vi "Power Supply Initialize Chain.vi"(0 "reference in":refnum<class "Power Supply.lvclass">, 5 "Power Supply Chain VISA Resource":refnum<visa-resource-name>="Serial-Hub-1", 7 "Baud Rate":u16(ring)=3 items=["1200", "2400", "4800", "9600", "19200"], 9 "Power Supply Chain Address (Master Unit)":i16=1, 11 "error in (no error)":errorcluster) -> (4 "reference out":refnum<class "Power Supply.lvclass">, 6 "PowerSupply Chain VISA Session":refnum<visa-resource-name>, 15 "error out":errorcluster)   [LabVIEW 2017, in "Power Supply.lvclass"]
uses:
  Power Supply.lvclass
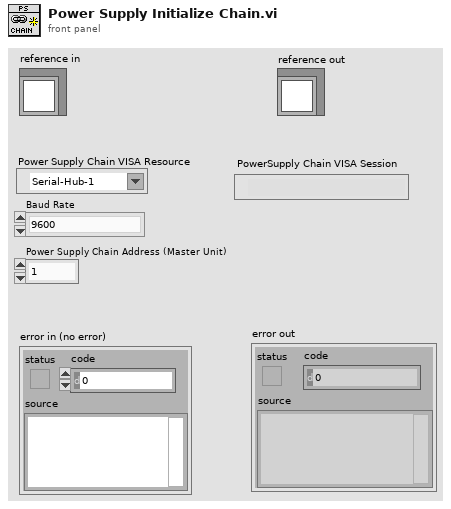
[diagram p1: front panel]
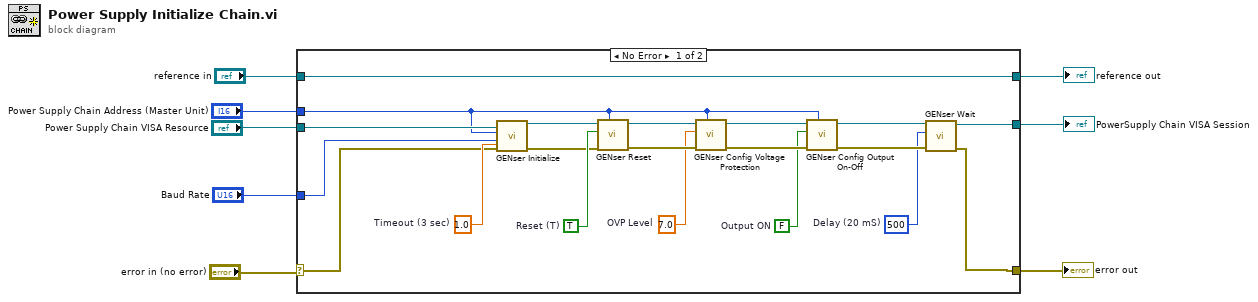
[diagram p0: block diagram]
diagram:
  n1 = case shown="No Error" "error in (no error)" {
    selector: "error in (no error)" -> [w13 w30]
    tunnel: [w10 w30] -> w7
    tunnel: "reference in" -> [w28 w29]
    tunnel: [w28 w29] -> w5
    tunnel: "Power Supply Chain VISA Resource" -> [w14 _]
    tunnel: [w12 _] -> w3
    tunnel: "Baud Rate" -> [w11 _]
    tunnel: "Power Supply Chain Address (Master Unit)" -> [w9 _]
    frame No Error {
      w15 = u32 500  # Delay (20 mS)
      w18 = FALSE  # Output ON
      w19 = 7.0  # OVP Level
      w25 = TRUE  # Reset (T)
      w27 = 1.0  # Timeout (3 sec)
      n2 = call <instrlib>:"GENser Initialize.vi"("Timeout (3 sec)"=w27, "error in (no error)"=w13, "BAUD"=w11, "GEN Addr"=w9, "VISA name"=w14) -> ("error out"=w24:errorcluster, "VISA out"=w26:refnum<visa-resource-name>)  [unwired: 5 in]
      n3 = call <instrlib>:"GENser Reset.vi"("GEN Addr"=w9, "error"=w24, "Reset (T)"=w25, "VISA"=w26) -> ("error out"=w22:errorcluster, "VISA out"=w23:refnum<visa-resource-name>)  [unwired: 6 in]
      n4 = call <instrlib>:"GENser Config Voltage Protection.vi"("GEN Addr"=w9, "error"=w22, "OVP Level"=w19, "VISA"=w23) -> ("error out"=w20:errorcluster, "VISA out"=w21:refnum<visa-resource-name>)  [unwired: 6 in]
      n5 = call <instrlib>:"GENser Config Output On-Off.vi"("GEN Addr"=w9, "error"=w20, "Output ON"=w18, "VISA"=w21) -> ("error out"=w16:errorcluster, "VISA out"=w17:refnum<visa-resource-name>)  [unwired: 6 in]
      n6 = call <instrlib>:"GENser Wait.vi"("error"=w16, "Delay (20 mS)"=w15, "VISA"=w17) -> ("error out"=w10:errorcluster, "VISA out"=w12:refnum<visa-resource-name>)  [unwired: 7 in]
    }
    frame Error {
    }
  }
  "error out" <- w7
  "reference out" <- w5
  "PowerSupply Chain VISA Session" <- w3
